vi "Sort Numeric String Array.vi"(11 "Array Values":string[](array[string])) -> (1 "Column Values for Sorting as String":string[](array[string]), 3 "Sorted Array Values":string[](array[string]))   [LabVIEW 2009]
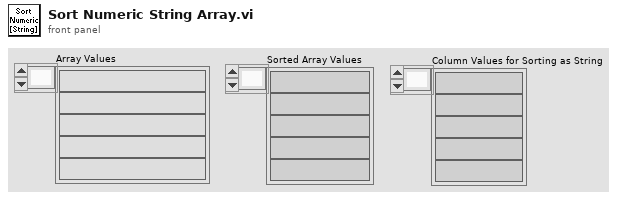
[diagram p1: front panel]
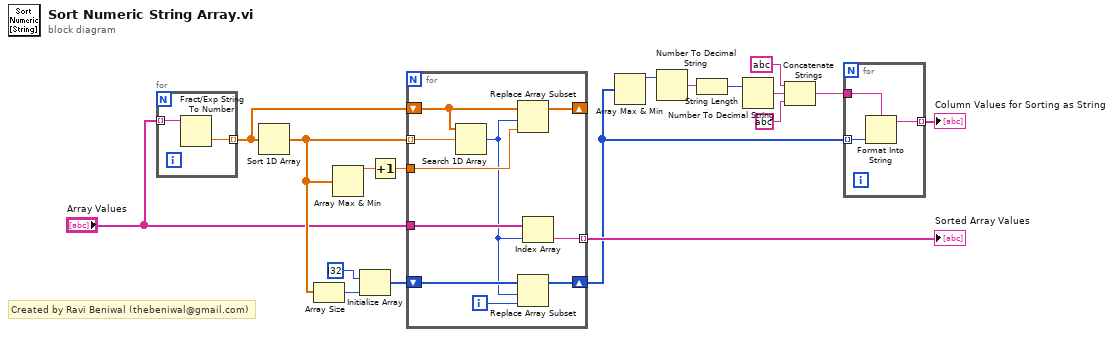
[diagram p0: block diagram]
diagram:
  # "Created by Ravi Beniwal (thebeniwal@gmail.com)"
  n1 = for {
    tunnel: "Array Values" -> [w19] mode=indexing
    tunnel: [w20] -> w3 mode=indexing
    n2 = Fract/Exp String To Number(string=w19) -> (number=w20:dbl)  [unwired: 3 in, 1 out]
  }
  n3 = Sort 1D Array(array=w3) -> (sorted array=w2:dbl[])
  n4 = Array Size(array=w2) -> (size(s)=w7:i32)
  n5 = Array Max & Min(array=w2) -> (max value=w18:dbl)  [unwired: 3 out]
  n6 = Initialize Array(i32 ?, w7) -> (w5:i32[])
  n7 = Increment(x=w18) -> (x+1=w17:dbl)
  n8 = for {
    tunnel: w2 -> [w30] mode=indexing
    shift-right: [w27] -> _
    shift-left: w3 -> [w29]
    tunnel: w17 -> [w28]
    tunnel: "Array Values" -> [w26]
    tunnel: [w25] -> w9 mode=indexing
    shift-right: [w23] -> w4
    shift-left: w5 -> [w24]
    i -> [w21]
    n9 = Search 1D Array(1D array=w29, element=w30) -> (index of element=w22:i32)  [unwired: 1 in]
    n10 = Replace Array Subset(array=w29, new element=w28, index=w22) -> (w27:dbl[])
    n11 = Replace Array Subset(array=w24, new element=w21, index=w22) -> (w23:i32[])
    n12 = Index Array(array=w26, index=w22) -> (element=w25:string)
  }
  "Sorted Array Values" <- w9
  n13 = Array Max & Min(array=w4) -> (max value=w15:i32)  [unwired: 3 out]
  n14 = Number To Decimal String(number=w15) -> (decimal integer string=w16:string)  [unwired: 1 in]
  n15 = String Length(string=w16) -> (length=w12:i32)
  n16 = Number To Decimal String(number=w12) -> (decimal integer string=w11:string)  [unwired: 1 in]
  n17 = Concatenate Strings(string ? ("format string"), w11, string ? ("format string")) -> (w10:string)
  n18 = for {
    tunnel: w4 -> [w33] mode=indexing
    tunnel: w10 -> [w32]
    tunnel: [w31] -> w8 mode=indexing
    n19 = Format Into String(format string=w32, w33) -> (resulting string=w31:string)  [unwired: 2 in, 1 out]
  }
  "Column Values for Sorting as String" <- w8
